vi "p5.2.vi"() -> ()   [LabVIEW 2020]
uses:
  <vilib>/Analysis/4window.llb/windowTd.ctl
  <vilib>/Analysis/3filter.llb/Filter Passband Type.ctl
  <vilib>/Analysis/NI_AALPro.lvlib
  <vilib>/Analysis/NI_AALBase.lvlib
panel:
  in  "low cutoff freq: fl":dbl
  in  "delta (rizado)":dbl=0.001 format="%#_13g"
  in  "Banda Transicion (normalizada)":dbl=0.1 format="%#_13g"
  out "N+1":i32=9
  out "DFT dB 2":dynamicdata(graph)
  out "DFT 2":dynamicdata(graph) caption="DFT"
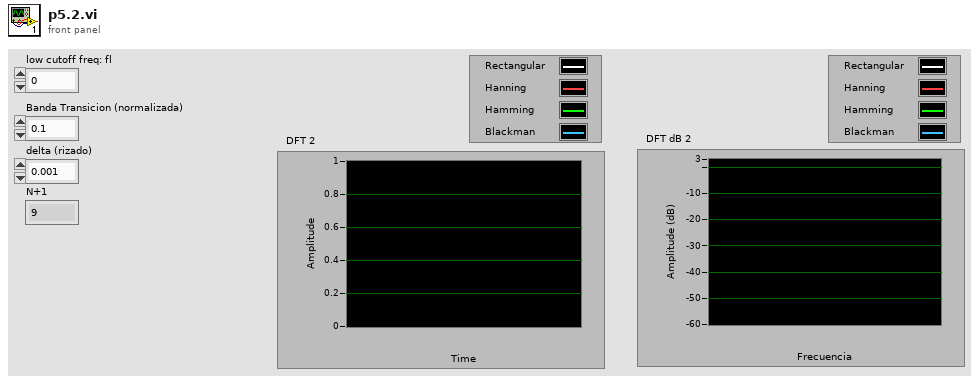
[diagram p1: front panel]
types:
  T1 = typedef "NI_AALBase.lvlib/Filter Passband Type.ctl" = enum32{"Lowpass", "Highpass", "Bandpass", "Bandstop"}
  T2 = typedef "NI_AALPro.lvlib/windowTd.ctl" = u32
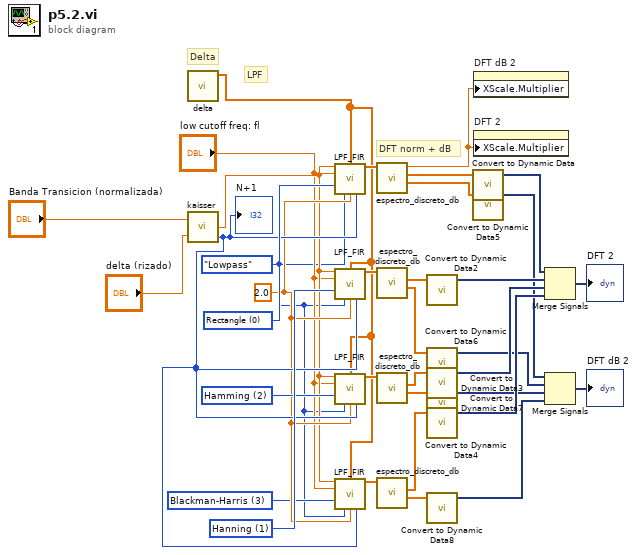
[diagram p0: block diagram]
diagram:
  w1 = Filter_Passband_Type."Lowpass" ("filter type")
  w6 = 2.0 ("sampling freq: fs")
  w5 = T2 3 items=["Rectangle"=0, "Hanning"=1, "Hamming"=2, "Blackman-Harris"=3, "Exact Blackman"=4, "Blackman"=5, "Flat Top"=6, "4 Term B-Harris "=7, "7 Term B-Harris"=8, "Low Sidelobe"=9, "Blackman Nuttall"=11, "Triangle"=30, "Bartlett-Hanning"=31, "Bohman"=32, "Parzen"=33, "Welch"=34, "Kaiser"=60, "Dolph-Chebyshev"=61, "Gaussian"=62] ("window")
  w9 = T2 2 items=["Rectangle"=0, "Hanning"=1, "Hamming"=2, "Blackman-Harris"=3, "Exact Blackman"=4, "Blackman"=5, "Flat Top"=6, "4 Term B-Harris "=7, "7 Term B-Harris"=8, "Low Sidelobe"=9, "Blackman Nuttall"=11, "Triangle"=30, "Bartlett-Hanning"=31, "Bohman"=32, "Parzen"=33, "Welch"=34, "Kaiser"=60, "Dolph-Chebyshev"=61, "Gaussian"=62] ("window")
  w12 = T2 1 items=["Rectangle"=0, "Hanning"=1, "Hamming"=2, "Blackman-Harris"=3, "Exact Blackman"=4, "Blackman"=5, "Flat Top"=6, "4 Term B-Harris "=7, "7 Term B-Harris"=8, "Low Sidelobe"=9, "Blackman Nuttall"=11, "Triangle"=30, "Bartlett-Hanning"=31, "Bohman"=32, "Parzen"=33, "Welch"=34, "Kaiser"=60, "Dolph-Chebyshev"=61, "Gaussian"=62] ("window")
  w14 = T2 0 items=["Rectangle"=0, "Hanning"=1, "Hamming"=2, "Blackman-Harris"=3, "Exact Blackman"=4, "Blackman"=5, "Flat Top"=6, "4 Term B-Harris "=7, "7 Term B-Harris"=8, "Low Sidelobe"=9, "Blackman Nuttall"=11, "Triangle"=30, "Bartlett-Hanning"=31, "Bohman"=32, "Parzen"=33, "Welch"=34, "Kaiser"=60, "Dolph-Chebyshev"=61, "Gaussian"=62] ("window")
  # "LPF"
  # "DFT norm + dB"
  # "Delta"
  n1 = call "delta.vi"() -> ("Array"=w2:dbl[])  [unwired: 11 in]
  n2 = call "kaisser.vi"("Banda Transicion (normalizada)"="Banda Transicion (normalizada)", "delta (rizado)"="delta (rizado)") -> ("Beta"=w4:dbl, "N+1"=w7:i32)  [unwired: 1 out]
  "N+1" <- w7
  n3 = call "LPF_FIR.vi"("window parameter"=w4, "Array"=w2, "low cutoff freq: fl"="low cutoff freq: fl", "window"=w14, "filter type"=w1, "sampling freq: fs"=w6, "taps"=w7) -> ("Filtered X"=w13:dbl[])  [unwired: 8 in]
  n4 = call "LPF_FIR.vi"("window parameter"=w4, "Array"=w2, "low cutoff freq: fl"="low cutoff freq: fl", "window"=w12, "filter type"=w1, "sampling freq: fs"=w6, "taps"=w7) -> ("Filtered X"=w11:dbl[])  [unwired: 8 in]
  n5 = call "LPF_FIR.vi"("window parameter"=w4, "Array"=w2, "low cutoff freq: fl"="low cutoff freq: fl", "window"=w9, "filter type"=w1, "sampling freq: fs"=w6, "taps"=w7) -> ("Filtered X"=w10:dbl[])  [unwired: 8 in]
  n6 = call "LPF_FIR.vi"("window parameter"=w4, "Array"=w2, "low cutoff freq: fl"="low cutoff freq: fl", "window"=w5, "filter type"=w1, "sampling freq: fs"=w6, "taps"=w7) -> ("Filtered X"=w8:dbl[])  [unwired: 8 in]
  n7 = call "espectro_discreto_db.vi"("Filtered X"=w13) -> ("DFT dB"=w27:dbl[], "DFT"=w35:dbl[], "Multiplier factor"=w17:dbl)  [unwired: 8 in]
  n8 = call "espectro_discreto_db.vi"("Filtered X"=w11) -> ("DFT dB"=w25:dbl[], "DFT"=w33:dbl[])  [unwired: 8 in, 1 out]
  n9 = call "espectro_discreto_db.vi"("Filtered X"=w10) -> ("DFT dB"=w23:dbl[], "DFT"=w31:dbl[])  [unwired: 8 in, 1 out]
  n10 = call "espectro_discreto_db.vi"("Filtered X"=w8) -> ("DFT dB"=w21:dbl[], "DFT"=w29:dbl[])  [unwired: 8 in, 1 out]
  n11 = call "Convert to Dynamic Data2"("Array"=w33) -> ("Dynamic Data Type"=w32:dynamicdata)  [unwired: 3 in]
  n12 = call "Convert to Dynamic Data6"("Array"=w25) -> ("Dynamic Data Type"=w24:dynamicdata)  [unwired: 3 in]
  n13 = call "Convert to Dynamic Data3"("Array"=w31) -> ("Dynamic Data Type"=w30:dynamicdata)  [unwired: 3 in]
  n14 = call "Convert to Dynamic Data7"("Array"=w23) -> ("Dynamic Data Type"=w22:dynamicdata)  [unwired: 3 in]
  n15 = call "Convert to Dynamic Data4"("Array"=w29) -> ("Dynamic Data Type"=w28:dynamicdata)  [unwired: 3 in]
  n16 = call "Convert to Dynamic Data8"("Array"=w21) -> ("Dynamic Data Type"=w20:dynamicdata)  [unwired: 3 in]
  n17 = call "Convert to Dynamic Data"("Array"=w35) -> ("Dynamic Data Type"=w34:dynamicdata)  [unwired: 3 in]
  n18 = call "Convert to Dynamic Data5"("Array"=w27) -> ("Dynamic Data Type"=w26:dynamicdata)  [unwired: 3 in]
  n19 = property on="DFT dB 2" class="WFGraph (strict)"("XScale.Multiplier"=w17) -> ()  [unwired: 2 in, 2 out]
  n20 = property on="DFT 2" class="WFGraph (strict)"("XScale.Multiplier"=w17) -> ()  [unwired: 2 in, 2 out]
  n21 = Merge Signals(w34, w32, w30, w28) -> (→"DFT 2":dynamicdata)
  n22 = Merge Signals(w26, w24, w22, w20) -> (→"DFT dB 2":dynamicdata)
